vi "Shut_down_Hi_Tecs.vi"(4 "Client Name":string) -> ()   [LabVIEW 2010]
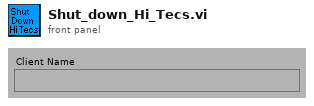
[diagram p1: front panel]
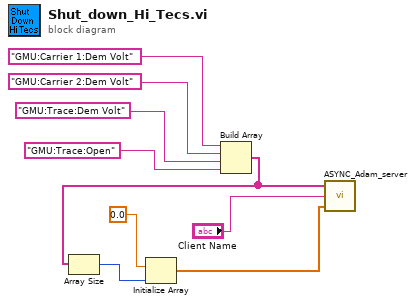
[diagram p0: block diagram]
diagram:
  n1 = Build Array("GMU:Carrier 1:Dem Volt", "GMU:Carrier 2:Dem Volt", "GMU:Trace:Dem Volt", "GMU:Trace:Open") -> (w4:string[])
  n2 = Array Size(array=w4) -> (size(s)=w5:i32)
  n3 = Initialize Array(0.0 ("element"), w5) -> (w2:dbl[])
  n4 = call "ASYNC_Adam_server.vi"("Values"=w2, "Client Name"="Client Name", "Channel Names"=w4) -> ()  [unwired: 3 out]
